vi "Configure Timebase.vi"   [LabVIEW 2016, in "Agilent 2000 3000 X-Series.lvlib"]
doc: "Configures timebase settings."
uses:
  Agilent 2000 3000 X-Series.lvlib
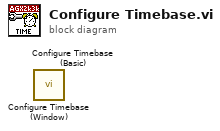
[diagram p0: block diagram]
diagram:
  n1 = call "Configure Timebase (Window).vi"() -> ()  [unwired: 14 in, 2 out]
  n2 = call "Configure Timebase (Basic).vi"() -> ()  [unwired: 14 in, 2 out]
